vi "Software Update HCC Update Software.vi"(5 "% Complete":refnum<vi>, 7 "Path Build List Sub":path[](array[path]), 8 "Error In":errorcluster, 9 "Update Files (Option 1-24) Sub":i32[](array[numeric]), 10 "Newfi Exe Folder Path":path=path "C:/Newfi Exe", 11 "New Software Location":path) -> (0 "Error Out":errorcluster)   [LabVIEW 2016]
panel:
  out "Current Location":path[](array[path])
  out "% Complete":u8(slide) scale=0.0..100.0
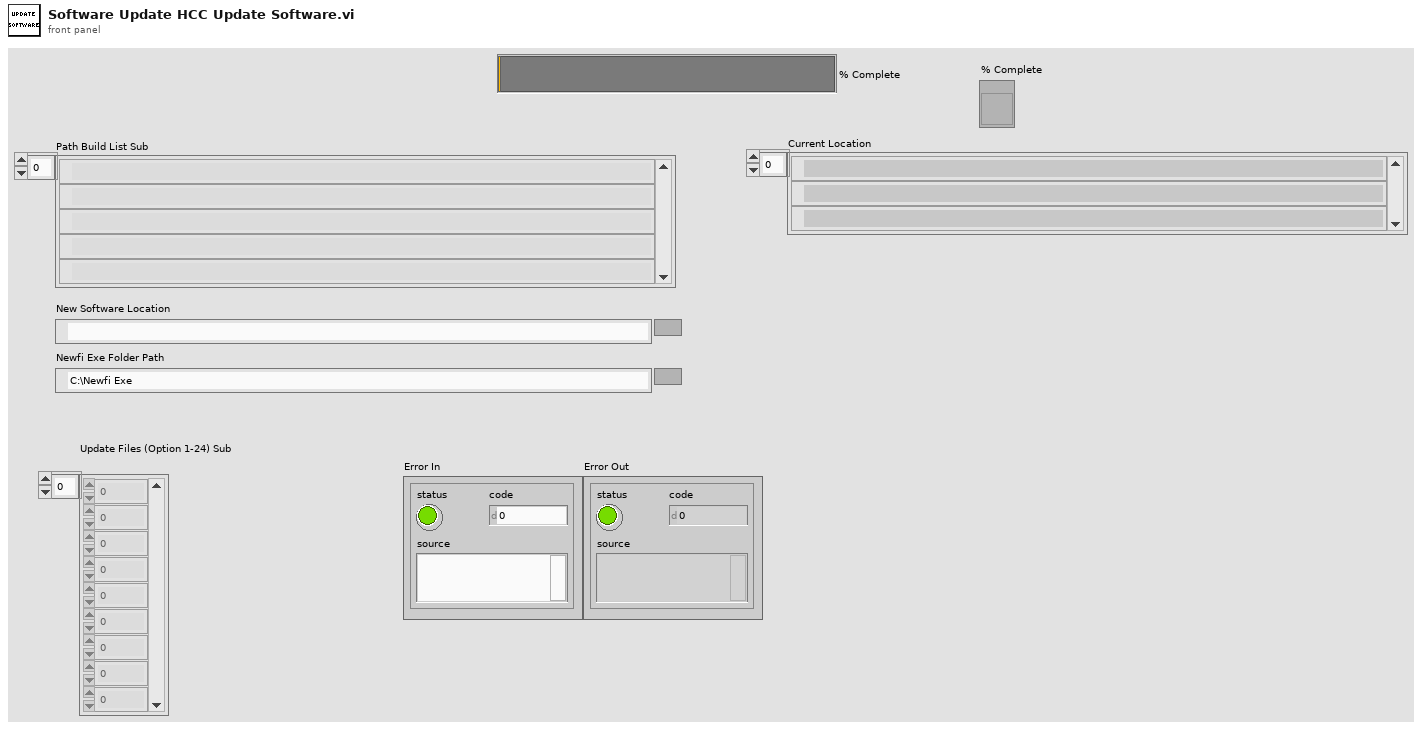
[diagram p1: front panel]
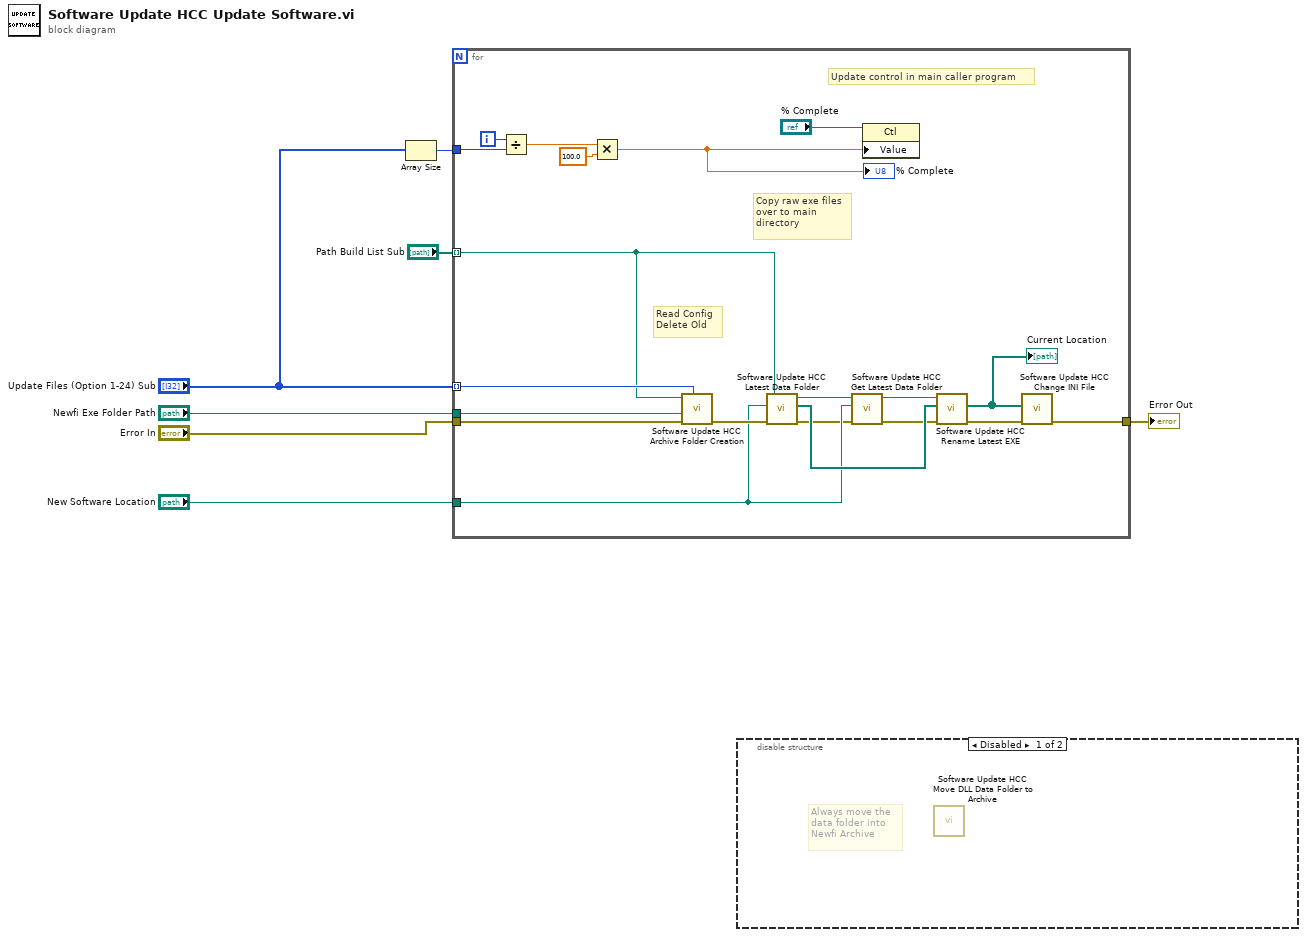
[diagram p0: block diagram]
diagram:
  n1 = Array Size(array="Update Files (Option 1-24) Sub") -> (size(s)=w7:i32)
  n2 = for {
    tunnel: "Path Build List Sub" -> [w20] mode=indexing
    tunnel: "Update Files (Option 1-24) Sub" -> [w21] mode=indexing
    tunnel: "New Software Location" -> [w13]
    tunnel: w7 -> [w26]
    tunnel: "Newfi Exe Folder Path" -> [w19]
    tunnel: "Error In" -> [w18]
    tunnel: [w10] -> w1
    i -> [w27]
    # "Copy raw exe files\nover to main \ndirectory"
    # "Read Config\nDelete Old"
    # "Update control in main caller program"
    n3 = Divide(x=w27, y=w26) -> (x/y=w25:dbl)
    n4 = Multiply(x=w25, y=100.0) -> (x*y=w23:dbl)
    "% Complete" <- w23
    n5 = call "Software Update HCC Archive Folder Creation.vi"("Numeric"=w21, "Error In"=w18, "Newfi Exe Folder Path"=w19, "Path Build List Sub"=w20) -> ("Error Out"=w15:errorcluster)  [unwired: 6 in, 1 out]
    n6 = call "Software Update HCC Latest Data Folder.vi"("error in (no error)"=w15, "New Software Location"=w13, "Path Build List Sub Input"=w20) -> ("error out"=w12:errorcluster, "Latest Exe Files"=w17:path[], "Path Build List Sub Output"=w14:path)  [unwired: 6 in]
    n7 = call "Software Update HCC Get Latest Data Folder.vi"("Error In"=w12, "New Software Location"=w13, "Path Build List Sub Input"=w14) -> ("Error Out"=w11:errorcluster, "Path Build List Sub Output"=w9:path)  [unwired: 7 in]
    n8 = property class="Ctl"(reference="% Complete", "Value"=w23) -> ()  [unwired: 1 in, 2 out]
    n9 = call "Software Update HCC Rename Latest EXE.vi"("error in (no error)"=w11, "Latest Exe Files"=w17, "Path Build List Sub Input"=w9) -> ("error out"=w16:errorcluster, "Array"=w8:path[])  [unwired: 7 in]
    "Current Location" <- w8
    n10 = call "Software Update HCC Change INI File.vi"("Error In"=w16, "Array"=w8) -> ("Error Out"=w10:errorcluster)  [unwired: 9 in]
  }
  "Error Out" <- w1
  n11 = disable-structure shown="Disabled" {
    frame Disabled {
      # "Always move the\ndata folder into\nNewfi Archive"
      n12 = call "Software Update HCC Move DLL Data Folder to Archive.vi"() -> ()  [unwired: 11 in, 1 out]
    }
    frame Enabled {
    }
  }
